vi "tm3samp_08_dcimgreader.vi"() -> ()   [LabVIEW 2011]
panel:
  out "Error Out":errorcluster
  out "Image":u16[][](graph)
  out "Time Stamp":dbl
  out "Total":i32
  in  "Index":i32 min=0 max=99 step=1
  out "Openfile":bool
  in  "Quit":bool
  in  "Open":bool
  in  "Frame Index":i32(c297)
  in  "DCIMG Path":path
  # "This is an example of how to read the images\nwithin a DCIMG file."
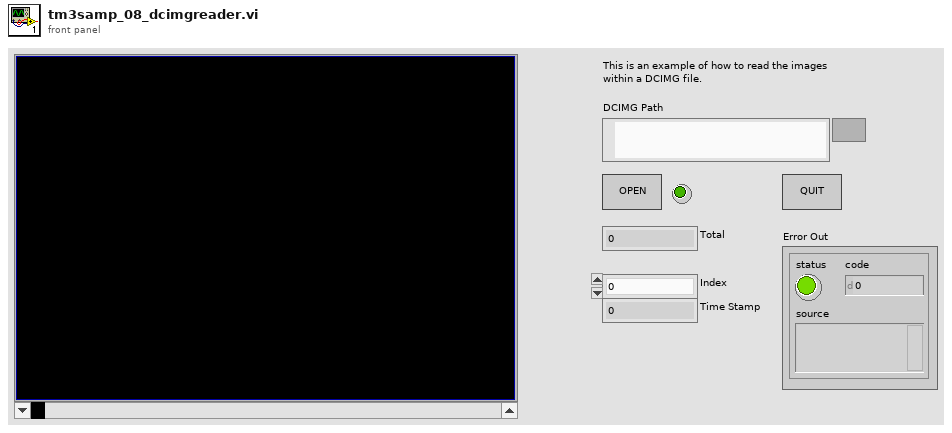
[diagram p1: front panel]
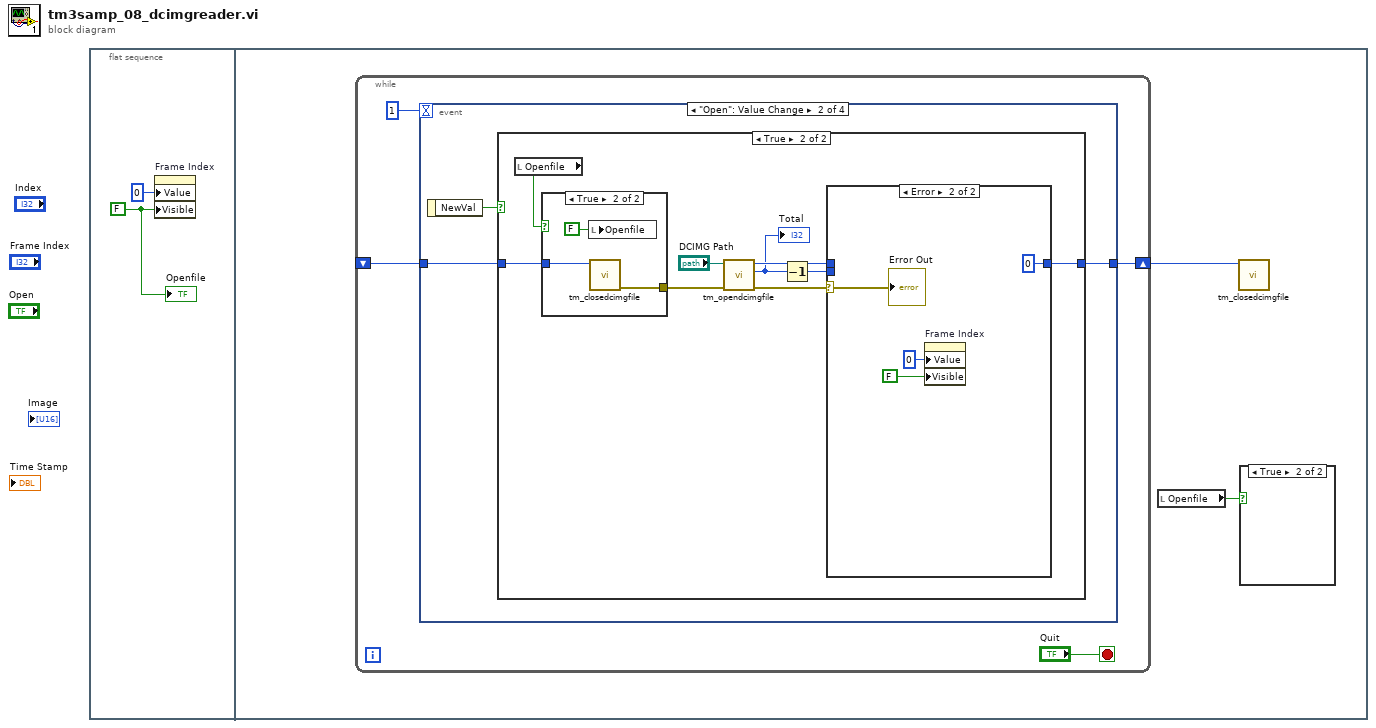
[diagram p0: block diagram]
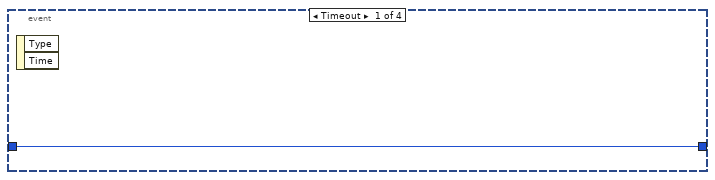
[diagram p3: hidden frame]
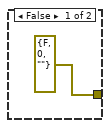
[diagram p5: hidden frame]
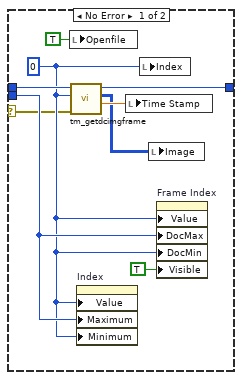
[diagram p6: hidden frame]
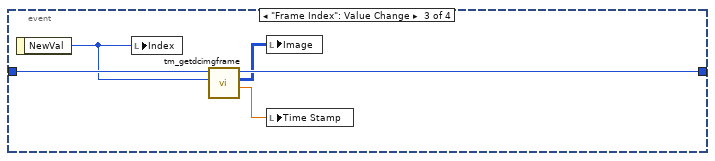
[diagram p7: hidden frame]
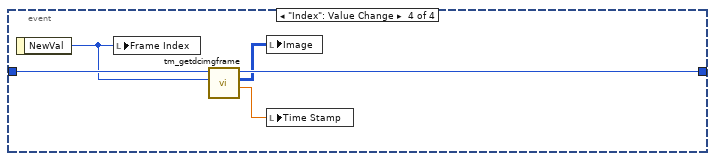
[diagram p8: hidden frame]
diagram:
  n1 = flat-sequence {
    frame #0 {
      w1 = FALSE ("Visible")
      n2 = property on="Frame Index" class="Scroll (strict)"("Value"=0 ("Frame Index"), "Visible"=w1) -> ()  [unwired: 2 in, 2 out]
      "Openfile" <- w1
    }
    frame #1 {
      n3 = while {
        shift-right: [w8] -> w3
        shift-left: _ -> [w7]
        stop <- "Quit" stop-if-true
        n4 = event shown="[1] \"Open\": Value Change" {
          selector: _ -> [_ _ _ _]
          dyn-events: _ -> [_ _ _ _]
          timeout: 1 -> [_ _ _ _]
          tunnel: [w9 w11 w43 w48] -> w8
          tunnel: w7 -> [w9 w10 w44 w49]
          event Timeout {
            n5 = event-data() -> ()  [unwired: 1 in, 2 out]
          }
          event "Open": Value Change {
            n6 = event-data() -> ("NewVal"=w12:bool)  [unwired: 1 in]
            n7 = case shown="True" w12 {
              tunnel: [w13 w20] -> w11
              tunnel: w10 -> [w13 w19]
              frame False {
              }
              frame True {
                n8 = local read "Openfile"() -> (w18:bool)
                n9 = case shown="True" w18 {
                  tunnel: w19 -> [_ w26]
                  tunnel: [errorcluster {"status"=FALSE, "code"=0, "source"=""} ("error out") w24] -> w17
                  frame False {
                  }
                  frame True {
                    n10 = local write "Openfile"(FALSE ("Openfile")) -> ()
                    n11 = call <userlib>:"tm_closedcimgfile.vi"("File Handle"=w26) -> ("error out"=w24:errorcluster)  [unwired: 10 in]
                  }
                }
                n12 = call <userlib>:"tm_opendcimgfile.vi"("error in (no error)"=w17, "Path"="DCIMG Path") -> ("error out"=w16:errorcluster, "Total Frames"=w15:i32, "File Handle"=w21:u32)  [unwired: 7 in]
                "Total" <- w15
                n13 = Decrement(x=w15) -> (x-1=w14:i32)
                n14 = case shown="Error" w16 {
                  selector: w16 -> [w28 w36]
                  tunnel: w21 -> [w35 _]
                  tunnel: w14 -> [w30 _]
                  tunnel: [w34 u32 0 ("File Handle out")] -> w20
                  frame No Error {
                    w29 = 0 ("Frame Index")
                    n15 = local write "Openfile"(TRUE ("Openfile")) -> ()
                    n16 = call <userlib>:"tm_getdcimgframe.vi"("error in (no error)"=w28, "Frame Index"=w29, "File Handle in"=w35) -> ("Time Sec"=w31:dbl, "Data"=w27:u16[][], "File Handle out"=w34:u32)  [unwired: 5 in, 1 out]
                    n17 = property on="Index" class="DigNum (strict)"("Value"=w29, "Maximum"=w30, "Minimum"=w29) -> ()  [unwired: 2 in, 2 out]
                    n18 = local write "Time Stamp"(w31) -> ()
                    n19 = local write "Index"(w29) -> ()
                    n20 = local write "Image"(w27) -> ()
                    n21 = property on="Frame Index" class="Scroll (strict)"("Value"=w29, "DocMax"=w30, "DocMin"=w29, "Visible"=TRUE) -> ()  [unwired: 2 in, 2 out]
                  }
                  frame Error {
                    n22 = property on="Frame Index" class="Scroll (strict)"("Value"=0 ("Frame Index"), "Visible"=FALSE) -> ()  [unwired: 2 in, 2 out]
                    "Error Out" <- w36
                  }
                }
              }
            }
          }
          event "Frame Index": Value Change {
            n23 = event-data() -> ("NewVal"=w42:i32)  [unwired: 1 in]
            n24 = local write "Index"(w42) -> ()
            n25 = call <userlib>:"tm_getdcimgframe.vi"("Frame Index"=w42, "File Handle in"=w44) -> ("Time Sec"=w40:dbl, "Data"=w41:u16[][], "File Handle out"=w43:u32)  [unwired: 6 in, 1 out]
            n26 = local write "Image"(w41) -> ()
            n27 = local write "Time Stamp"(w40) -> ()
          }
          event "Index": Value Change {
            n28 = event-data() -> ("NewVal"=w47:i32)  [unwired: 1 in]
            n29 = local write "Frame Index"(w47) -> ()
            n30 = call <userlib>:"tm_getdcimgframe.vi"("Frame Index"=w47, "File Handle in"=w49) -> ("Time Sec"=w45:dbl, "Data"=w46:u16[][], "File Handle out"=w48:u32)  [unwired: 6 in, 1 out]
            n31 = local write "Image"(w46) -> ()
            n32 = local write "Time Stamp"(w45) -> ()
          }
        }
      }
      n33 = local read "Openfile"() -> (w4:bool)
      n34 = call <userlib>:"tm_closedcimgfile.vi"("File Handle"=w3) -> ()  [unwired: 10 in, 1 out]
      n35 = case shown="True" w4 {
        frame False {
        }
        frame True {
        }
      }
    }
  }
